vi "Create Payload (Increment).vi"(7 "Bit Length":u16(ring) items=["Byte (8 bits)", "Word (16 bits)", "Long (32 bits)", "Quad (64 bits)"], 9 "Interval":u64 format="%.0x", 10 "Start Value":u64 format="%.0x", 11 "Length":i32) -> (2 "Value not in range?":bool, 3 "Payload (U8)":u8[](array[numeric]) format="%.0x")   [LabVIEW 2020, in "EthFrameManagement.lvlib"]
uses:
  EthFrameManagement.lvlib
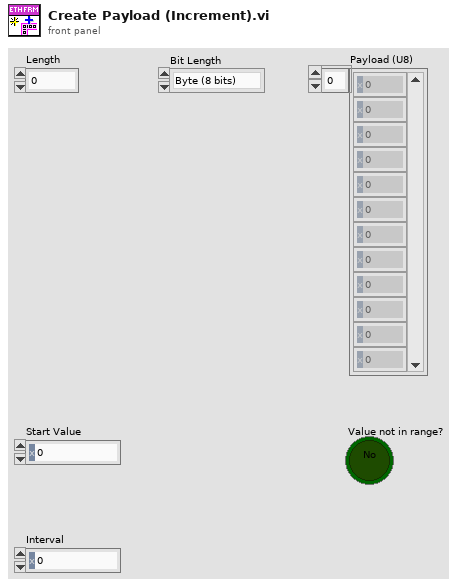
[diagram p1: front panel]
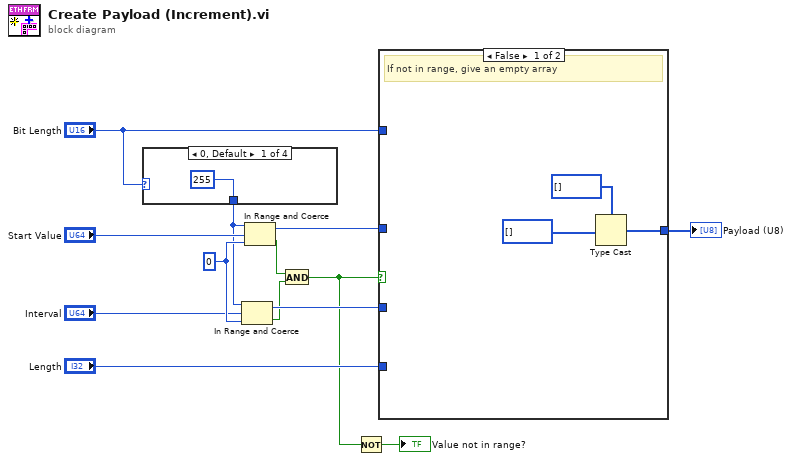
[diagram p0: block diagram]
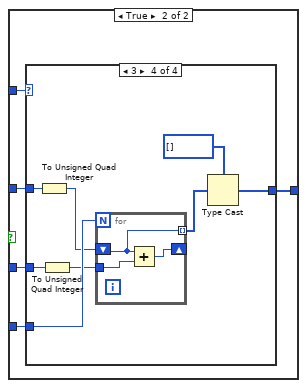
[diagram p2: hidden frame]
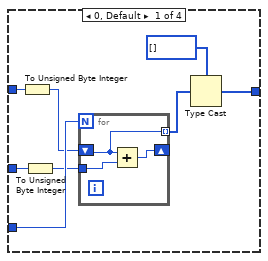
[diagram p3: hidden frame]
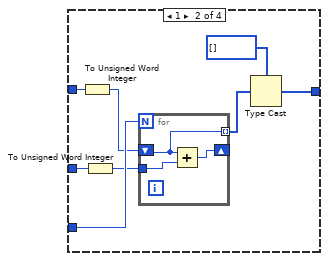
[diagram p4: hidden frame]
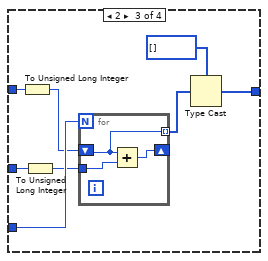
[diagram p5: hidden frame]
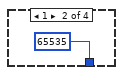
[diagram p6: hidden frame]
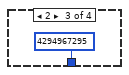
[diagram p7: hidden frame]
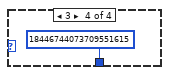
[diagram p8: hidden frame]
diagram:
  w6 = u64 0 ("lower limit")
  n1 = case shown="0, Default" "Bit Length" {
    tunnel: [u64 255 ("upper limit") u64 65535 ("upper limit") u64 4294967295 ("upper limit") u64 18446744073709551615 ("upper limit")] -> w4
    frame 0, Default {
    }
    frame 1 {
    }
    frame 2 {
    }
    frame 3 {
    }
  }
  n2 = In Range and Coerce(upper limit=w4, x="Interval", lower limit=w6) -> (coerced(x)=w3:u64, In Range?=w1:bool)
  n3 = In Range and Coerce(upper limit=w4, x="Start Value", lower limit=w6) -> (coerced(x)=w11:u64, In Range?=w9:bool)
  n4 = And(x=w9, y=w1) -> (x .and. y?=w2:bool)
  n5 = Not(x=w2) -> (.not. x?=→"Value not in range?":bool)
  n6 = case shown="False" w2 {
    tunnel: "Bit Length" -> [_ w25]
    tunnel: w11 -> [_ w24]
    tunnel: "Length" -> [_ w23]
    tunnel: [w19 w22] -> w8
    tunnel: w3 -> [_ w21]
    frame False {
      # "If not in range, give an empty array"
      n7 = Type Cast(type=u8[] [] ("Array"), x=u8[] [] ("Array")) -> (*(type *) &x=w19:u8[])
    }
    frame True {
      n8 = case shown="3" w25 {
        tunnel: w24 -> [w33 w44 w55 w66]
        tunnel: w23 -> [w30 w41 w52 w63]
        tunnel: [w31 w42 w53 w64] -> w22
        tunnel: w21 -> [w29 w40 w51 w62]
        frame 0, Default {
          n9 = To Unsigned Byte Integer(number=w33) -> (unsigned 8bit integer=w28:u8)
          n10 = To Unsigned Byte Integer(number=w29) -> (unsigned 8bit integer=w27:u8)
          n11 = for {
            N: w30 -> [_]
            tunnel: w27 -> [w36]
            tunnel: [w34] -> w26 mode=indexing
            shift-right: [w35] -> _
            shift-left: w28 -> [w34]
            n12 = Add(x=w34, y=w36) -> (x+y=w35:u8)
          }
          n13 = Type Cast(type=u8[] [] ("Array"), x=w26) -> (*(type *) &x=w31:u8[])
        }
        frame 1 {
          n14 = To Unsigned Word Integer(number=w44) -> (unsigned 16bit integer=w39:u16)
          n15 = To Unsigned Word Integer(number=w40) -> (unsigned 16bit integer=w38:u16)
          n16 = for {
            N: w41 -> [_]
            tunnel: w38 -> [w47]
            tunnel: [w45] -> w37 mode=indexing
            shift-right: [w46] -> _
            shift-left: w39 -> [w45]
            n17 = Add(x=w45, y=w47) -> (x+y=w46:u16)
          }
          n18 = Type Cast(type=u8[] [] ("Array"), x=w37) -> (*(type *) &x=w42:u8[])
        }
        frame 2 {
          n19 = To Unsigned Long Integer(number=w55) -> (unsigned 32bit integer=w50:u32)
          n20 = To Unsigned Long Integer(number=w51) -> (unsigned 32bit integer=w49:u32)
          n21 = for {
            N: w52 -> [_]
            tunnel: w49 -> [w58]
            tunnel: [w56] -> w48 mode=indexing
            shift-right: [w57] -> _
            shift-left: w50 -> [w56]
            n22 = Add(x=w56, y=w58) -> (x+y=w57:u32)
          }
          n23 = Type Cast(type=u8[] [] ("Array"), x=w48) -> (*(type *) &x=w53:u8[])
        }
        frame 3 {
          n24 = To Unsigned Quad Integer(1:w66) -> (0:w61:u64)
          n25 = To Unsigned Quad Integer(1:w62) -> (0:w60:u64)
          n26 = for {
            N: w63 -> [_]
            tunnel: w60 -> [w69]
            tunnel: [w67] -> w59 mode=indexing
            shift-right: [w68] -> _
            shift-left: w61 -> [w67]
            n27 = Add(x=w67, y=w69) -> (x+y=w68:u64)
          }
          n28 = Type Cast(type=u8[] [] ("Array"), x=w59) -> (*(type *) &x=w64:u8[])
        }
      }
    }
  }
  "Payload (U8)" <- w8
